vi "set lable top.vi"() -> ()   [LabVIEW 2009]
uses:
  Global/Global 1.vi
panel:
  out "read string":string
  in  "string to write":string="Q77,14\n"
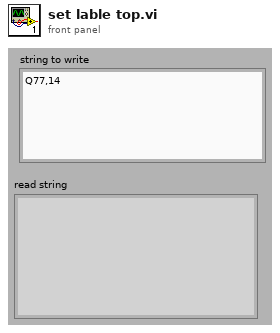
[diagram p1: front panel]
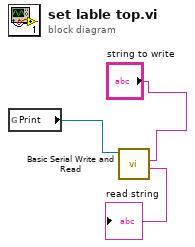
[diagram p0: block diagram]
diagram:
  n1 = global read "Global 1.vi" "Print"() -> (w3:refnum<visa-resource-name>)
  n2 = call "Basic Serial Write and Read.vi"("VISA resource name"=w3, "string to write"="string to write") -> ("read string"=→"read string":string)  [unwired: 7 in, 1 out]
